vi "diffraction pattern v2.0.vi"() -> ()   [LabVIEW 2019]
doc: "1. before run, set the paramaters on the left of the screen.\n2. flux (magnetic field) is in unit of flux quanta.\n3. Phaserange is in the unit of Pi, the CPR will be build up according to phase range of [-Phaserange/2,Phaserang/2], and such CPR will be a periodic function with Phaserange as period. Enter integer number of multiple times of 4 is preferred.\n4. Use the step setting tab to set resolution of the calculation, you can set how many points is used to define the width of the Josephson junction, how many points to represent the Phaserange\n5. Then you can choose which type of the CPR is used.\n6. Depending on the choose of the CPR, you may want to set the strength of the MBS, \"a\" parameter, the width of the gaussian function used, and the pattern of parity of MBS. Parity pattern has to have same number of elements for positive and negative range.\nEnter the parity 1 or -1 for positive and negative phase +-Pi, +-3Pi, +-5Pi etc.. in to the two arrays.\n7. You can use the index control to read the array elements, then enter the value, you can also delete an element of array by right click, the number of array elements is not limited.\n8. You can change the x,y range, zoom, create cursor etc. to help analyse the plot. Right click to save the data into excel.\n\nEnjoy!\nGuang Yue"
uses:
  dllparameter.ctl
  S-TI-S jj simulation c/Release/ygDLL.dll
panel:
  in  "Tab Control":T1(tab)
  in  "flux start":dbl=-5.0
  in  "flux end":dbl=5.0
  in  "flux step":dbl=0.1
  in  "Geometry steps":i32=201
  in  "Phase steps":i32=201
  in  "CPR Type":T2(ring)
  in  "CPR plot points":i32=500
  in  "parity for negative phase":i32[](array[numeric])=[1, -1, -1, 1]
  in  "Strenth of MBS":dbl=0.5
  in  "parity for positive phase":i32[](array[numeric])=[1, -1, 1, 1]
  in  "Gaussian width":dbl=0.2
  in  "Plot CPR":bool
  in  "Set Noise":bool
  out "Actual flux":dbl
  in  "Flux":dbl
  in  "Plot choice":enum32{"Icp", "Icn"}(radio)
  in  "Geometry Disorder Type":u16(ring) items=["Disorder OFF", "Disorder ON"]
  in  "Plot J vs y":bool
  out "error out":errorcluster
  in  "clear cpr":bool
  in  "clear j":bool
  in  "clearIc":bool
  out "Negative Phase0":dbl
  out "phaserange in Pi":i32=16
  out "Positive Phase0":dbl
  in  "Plot tab":T3(tab)
  out "Diffraction pattern plot":cluster{cluster{dbl, "icn":dbl}[]}[](graph)
  out "Phase0 vs Flux":cluster{cluster{dbl, "icn":dbl}[]}[](graph)
  out "J vs y":cluster{cluster{dbl, "icn":dbl}[]}[](graph)
  out "CPR":cluster{cluster{dbl, "icn":dbl}[]}[](graph)
  in  "Save":bool
  in  "hold":bool=TRUE
  out "Current Flux":dbl=5.0
  out "Remaining steps":i32
  in  "Exit":bool
  in  "Run":bool
  out "Total time s":dbl=5.020437899999706 format="%#_5g"
  in  "stop":bool
  out "Ic negative":dbl=-0.0009989221220817583
  out "Ic positive":dbl=0.000998922122081775 format="%#_5f"
  # "Go to Help menu for instructions, \nor move your mouse cursor on the \nobject for some tip."
  # "Calculate Diffraction pattern"
  # "Version 2.0"
  # "Switch the Tab to choose Plots to save"
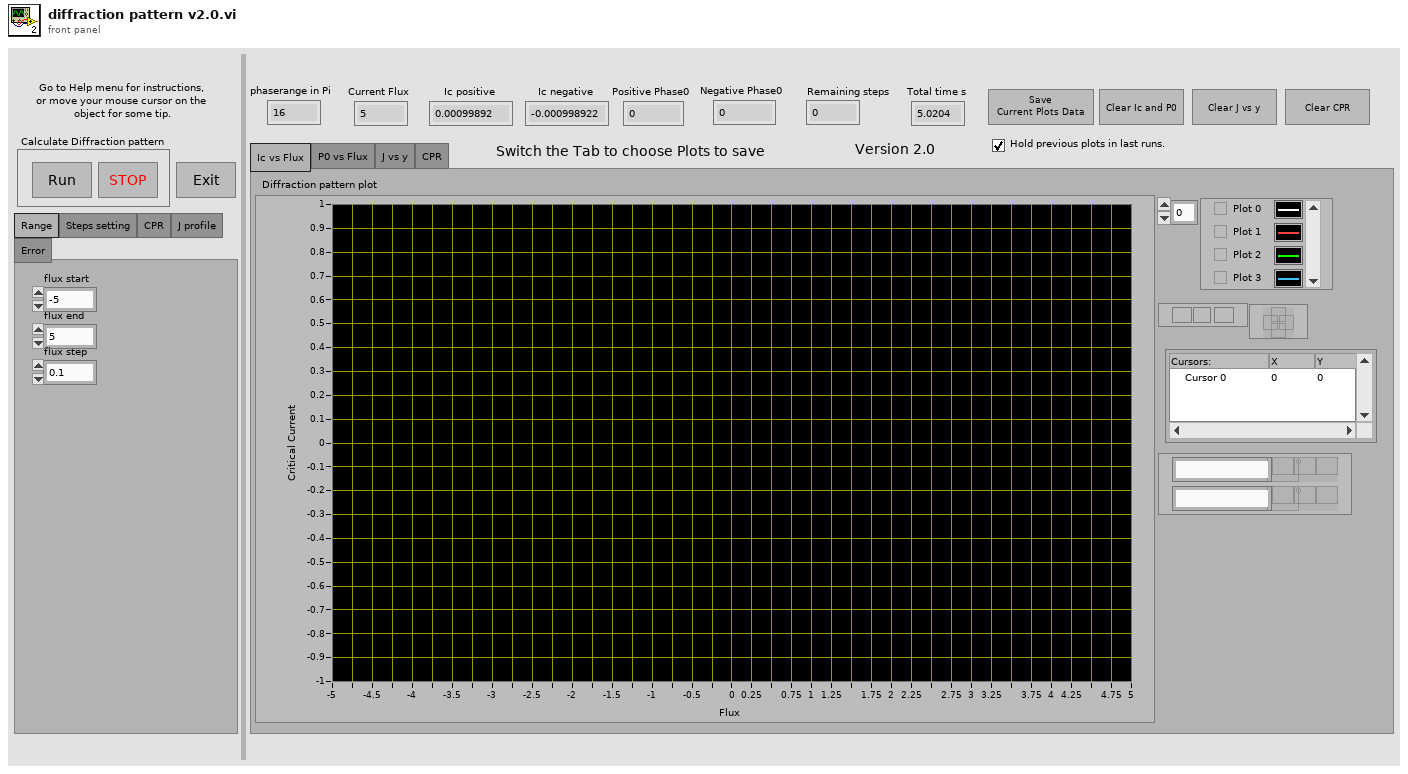
[diagram p1: front panel]
types:
  T1 = enum32{"Range", "Steps setting", "CPR", "J profile", "Error"}
  T2 = enum16{"Regular Josephson effect", "Non-local MBS", "Local MBS same parity", "Local MBS different parity"}
  T3 = enum32{"Ic vs Flux", "P0 vs Flux", "J vs y", "CPR"}
  T4 = enum32{"invalid app kind", "Development System", "Run Time System", "Student Edition", "Embedded LabVIEW", "Evaluation", "Custom"}
  T5 = enum8{"Enabled", "Disabled", "Disabled and Grayed Out"}
  T6 = typedef "dllparameter.ctl" = cluster{"parity for negative phase ":i32[], "parity for positive phase":i32[], "CPR Type":enum16{"Regular Josephson effect", "Non-local MBS", "Local MBS same parity", "Local MBS different parity"}, "Geometry Noise Type":u16, "Geometry steps":i32, "Phase steps":i32, "Strenth of MBS":dbl, "Gaussian width":dbl}
  T7 = cluster{cluster{"phase":dbl, "return type":dbl}[]}
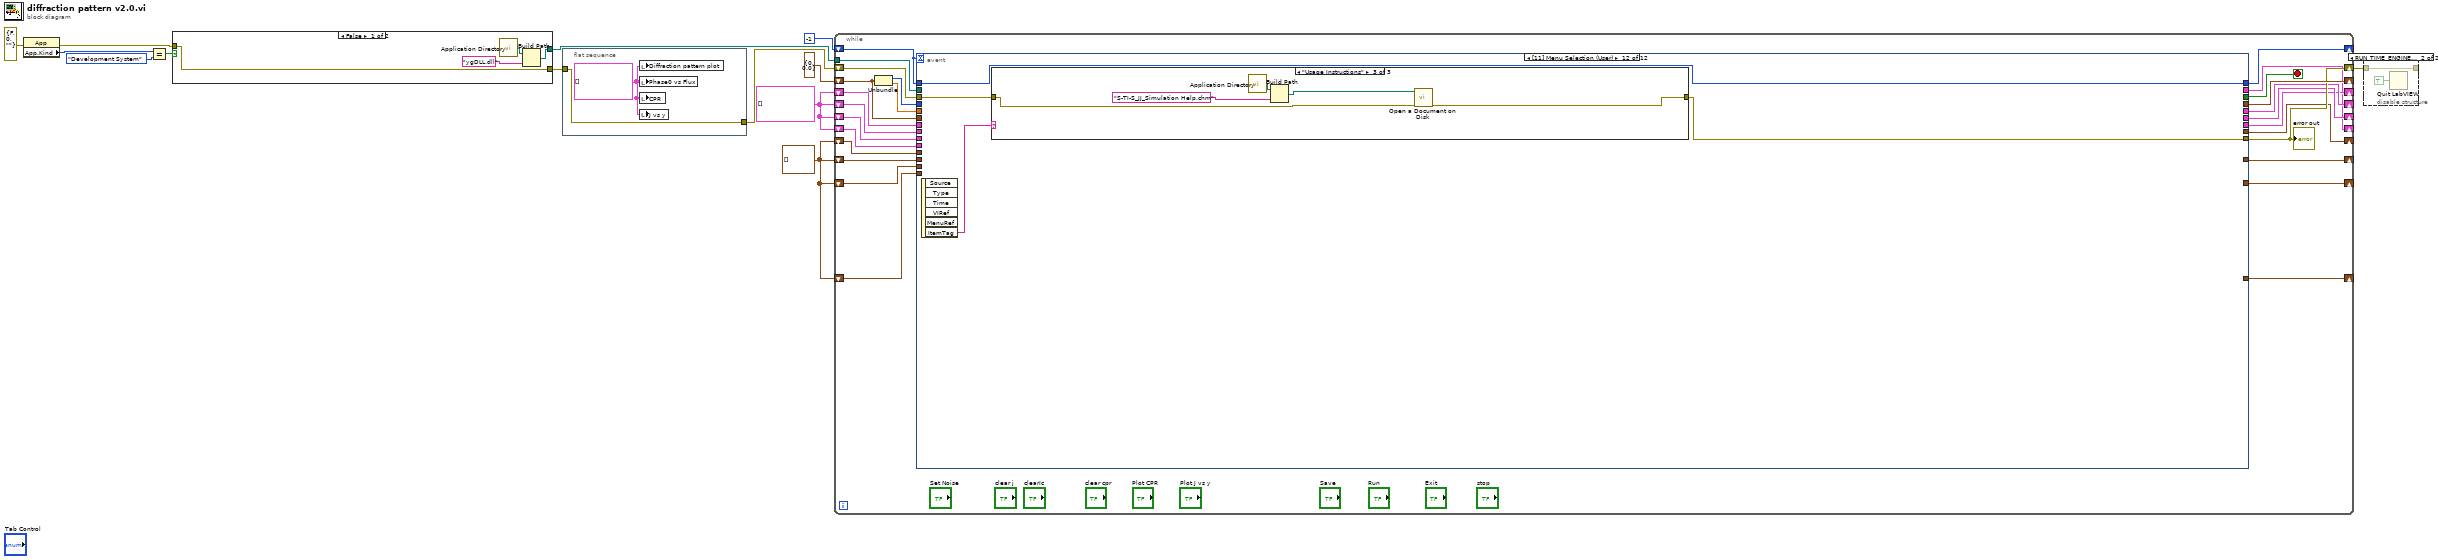
[diagram p0: block diagram]
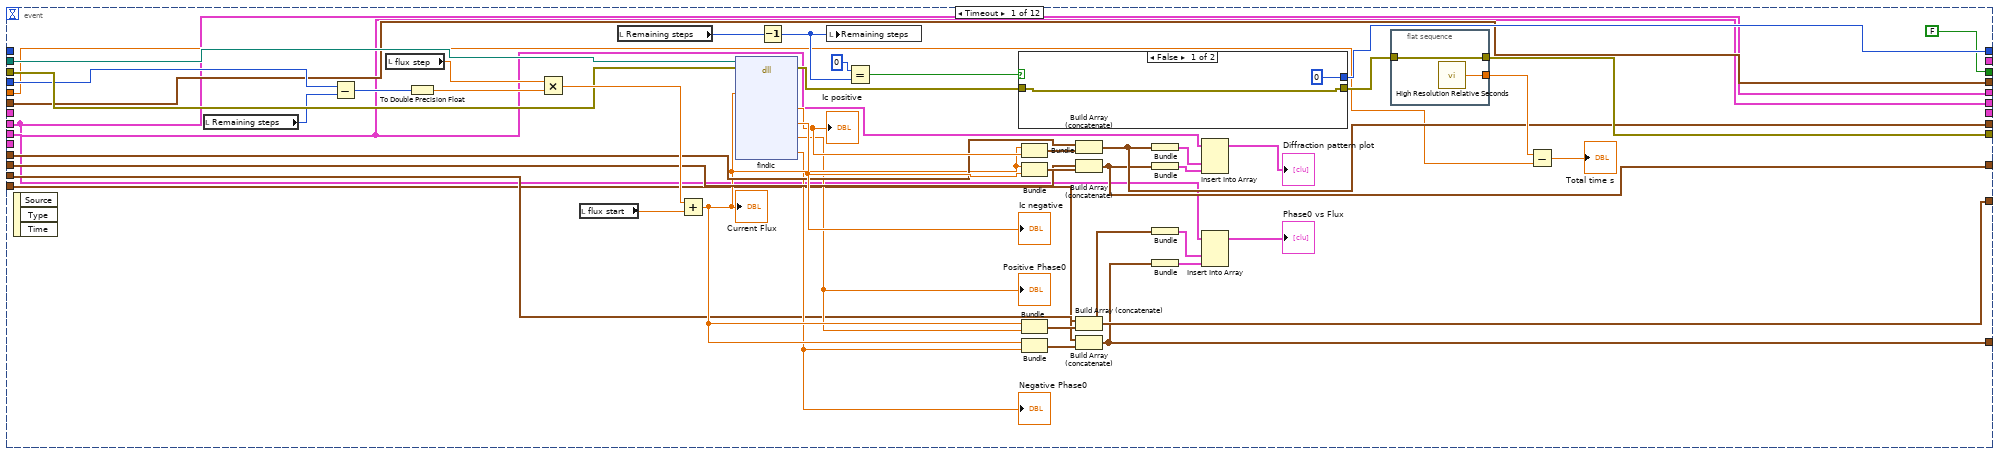
[diagram p3: hidden frame]
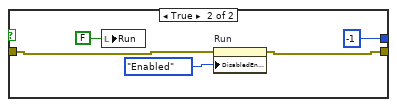
[diagram p4: hidden frame]
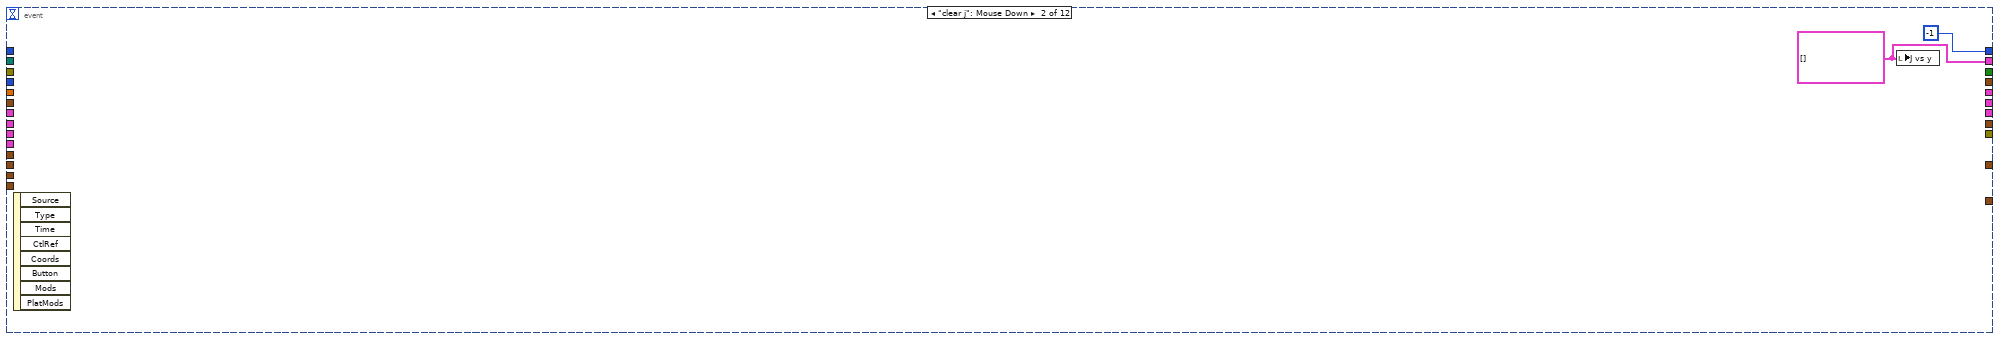
[diagram p5: hidden frame]
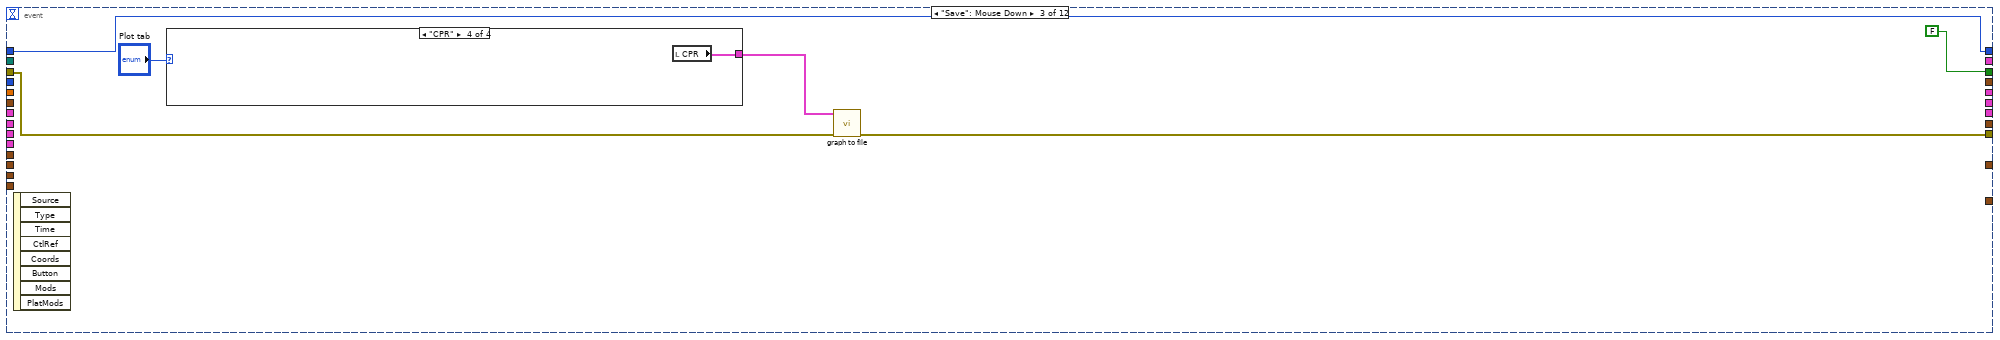
[diagram p6: hidden frame]
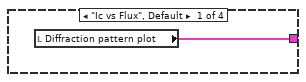
[diagram p7: hidden frame]
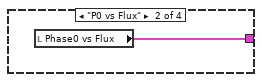
[diagram p8: hidden frame]
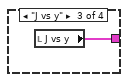
[diagram p9: hidden frame]
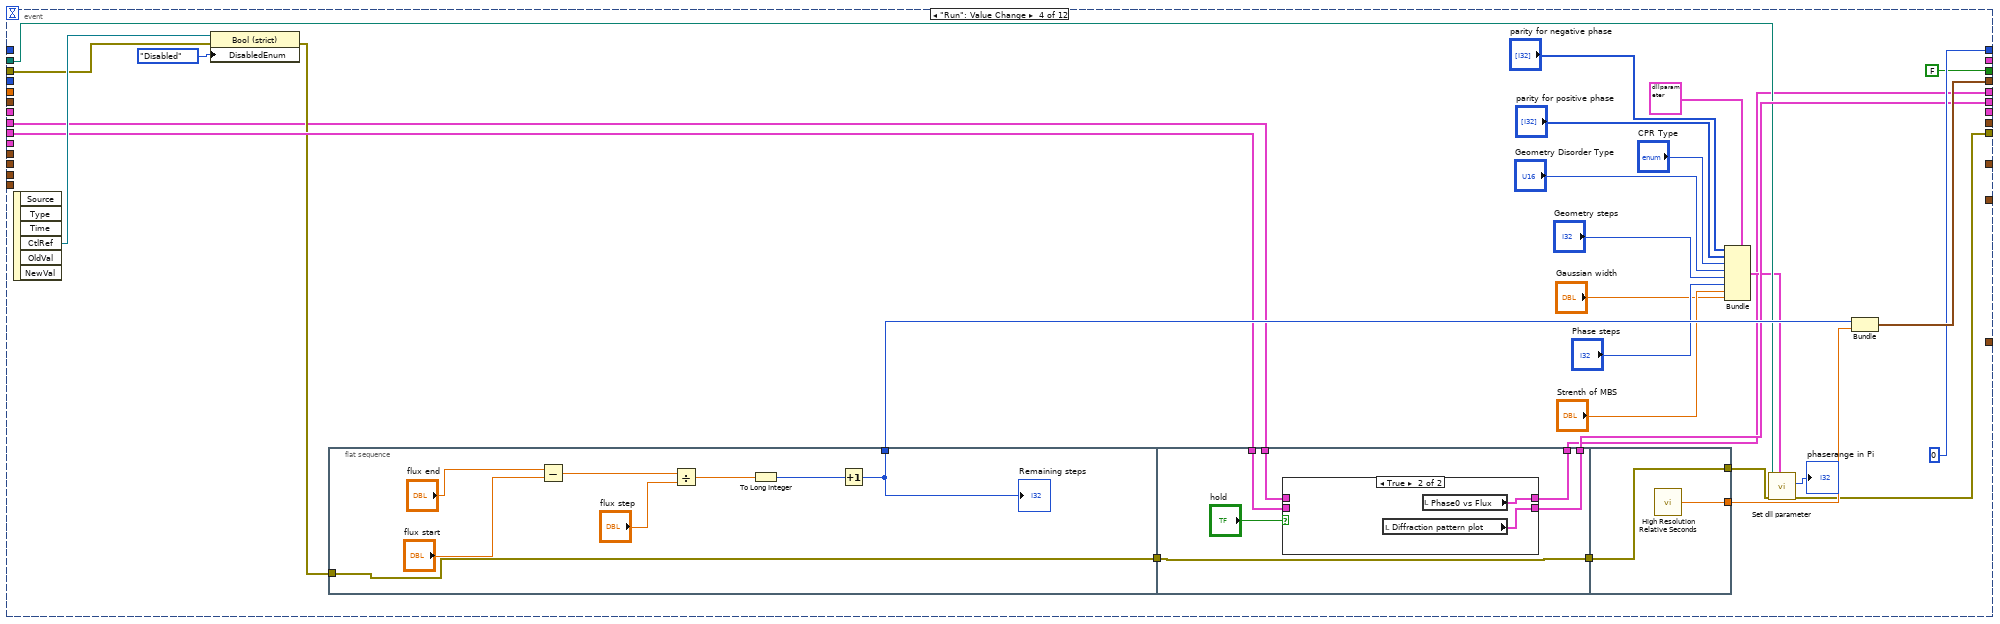
[diagram p10: hidden frame]
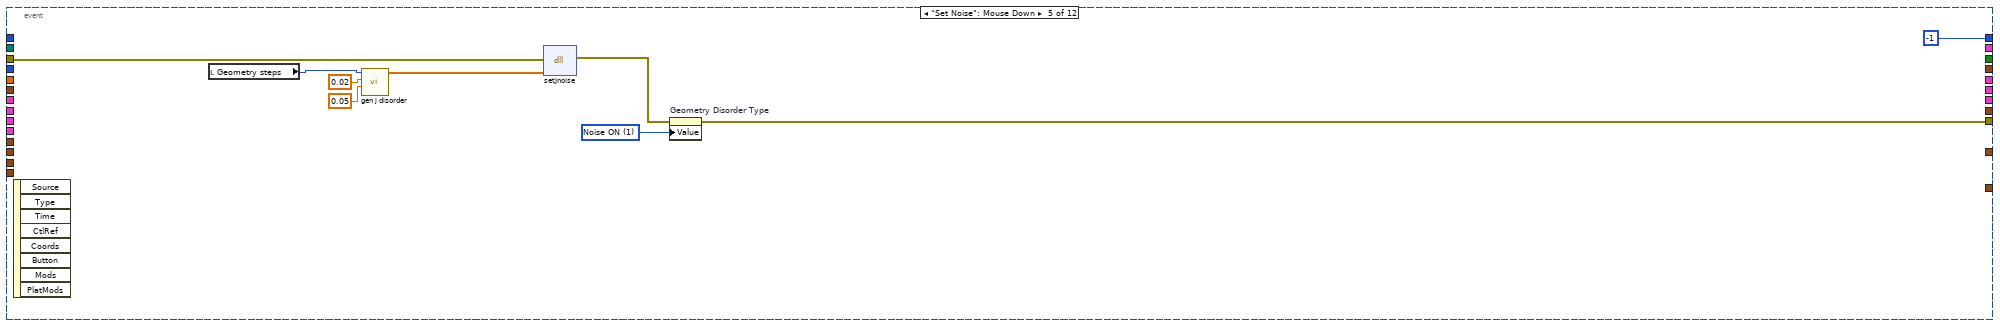
[diagram p12: hidden frame]
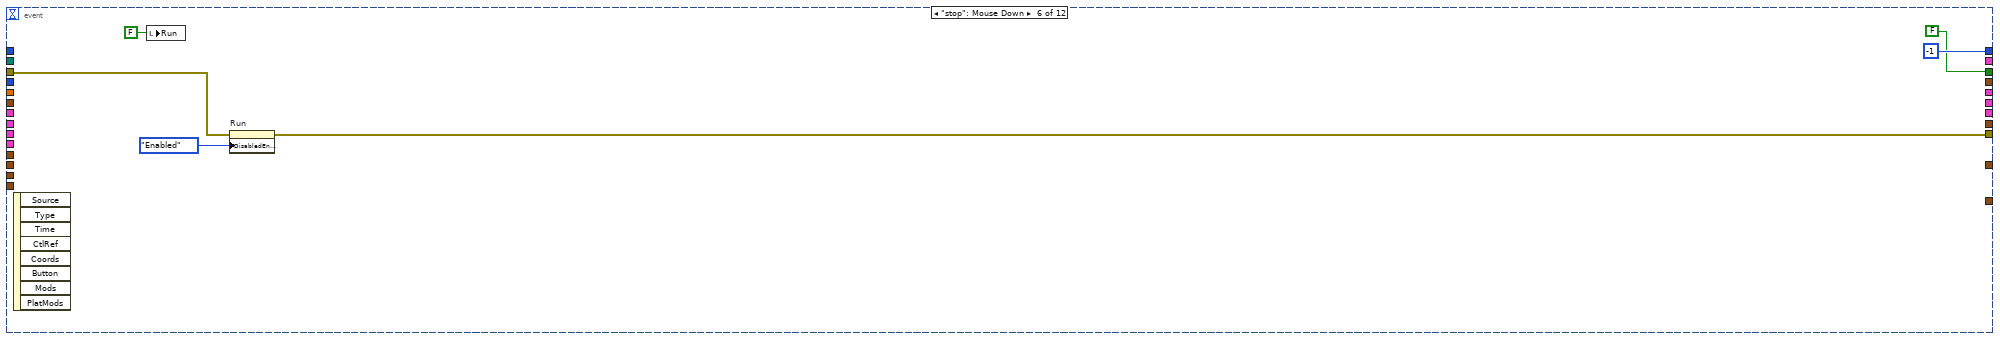
[diagram p13: hidden frame]
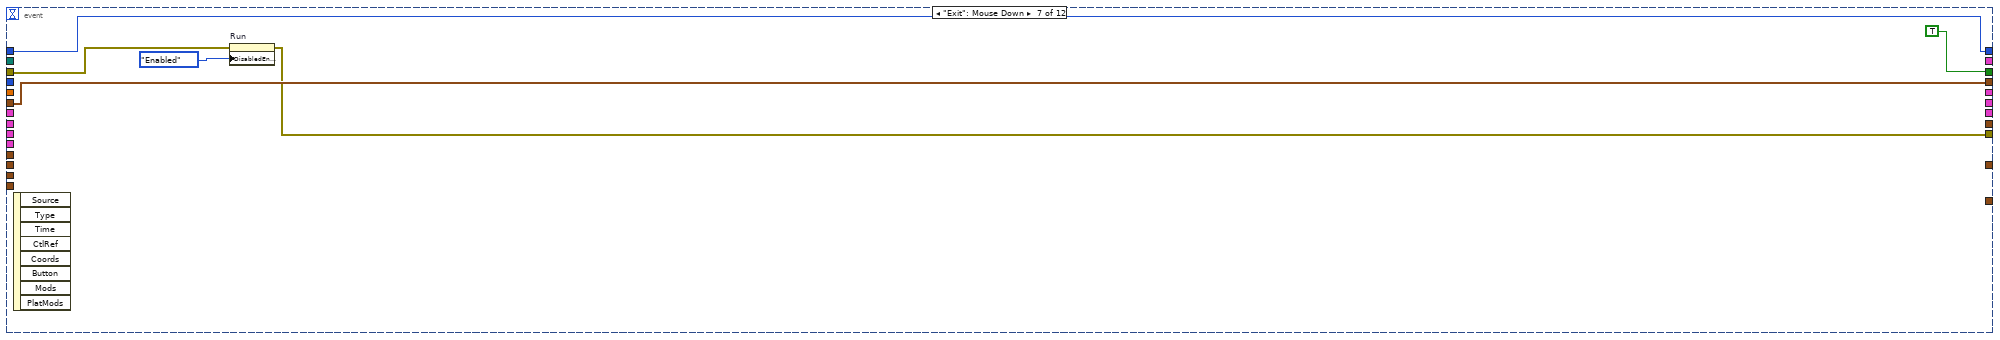
[diagram p14: hidden frame]
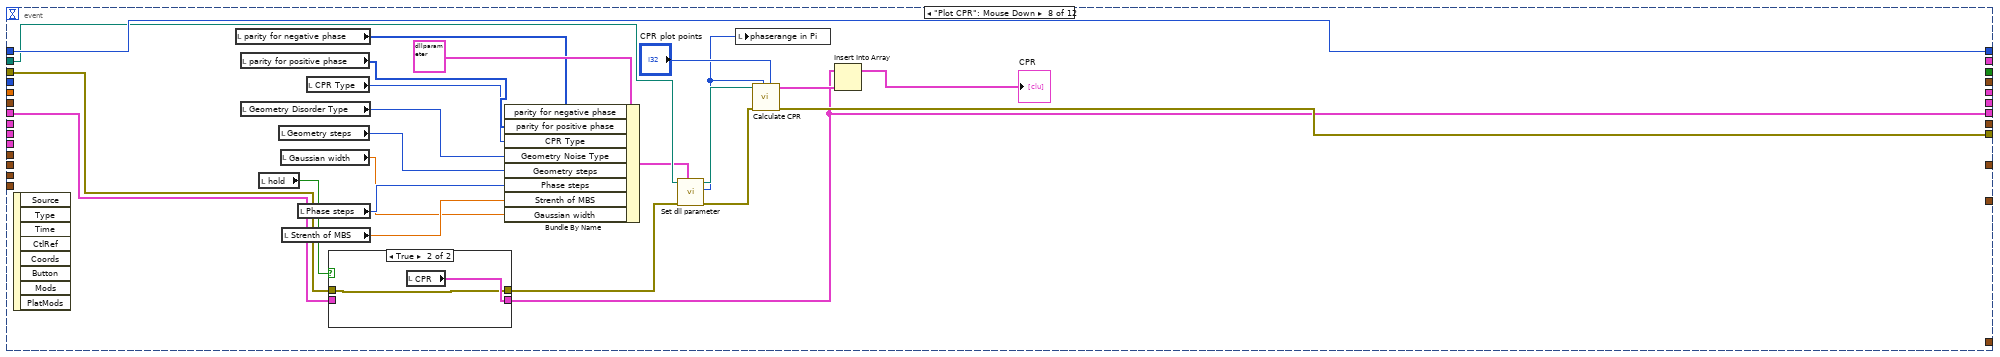
[diagram p15: hidden frame]
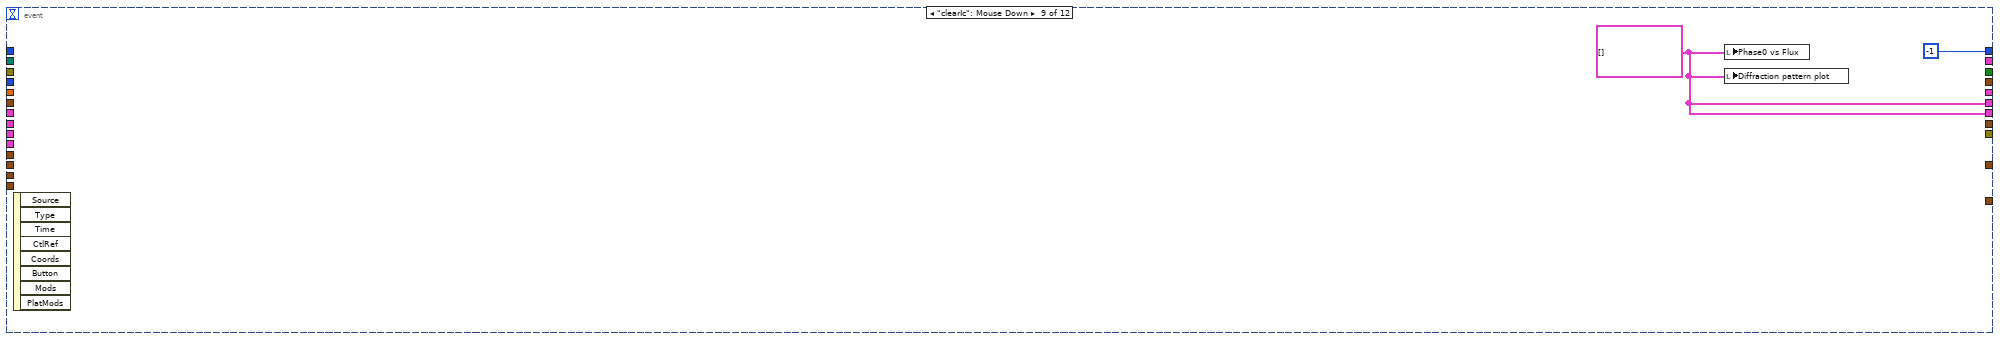
[diagram p17: hidden frame]
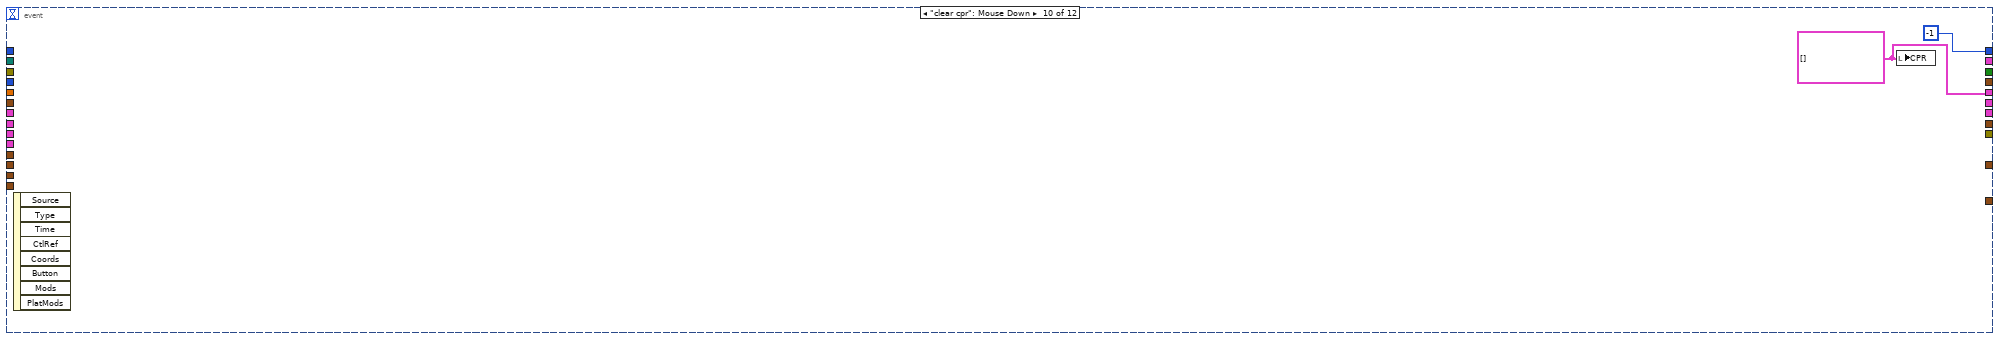
[diagram p18: hidden frame]
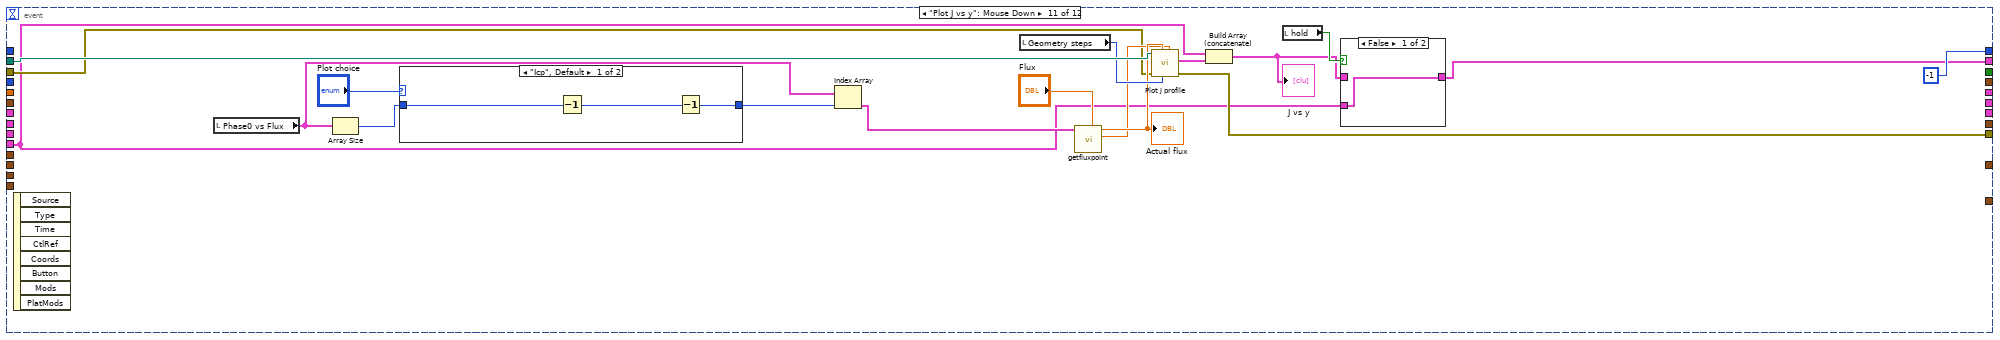
[diagram p19: hidden frame]
diagram:
  w1 = cluster{cluster{dbl, "icn":dbl}[]}[] [] ("appended array")
  w2 = cluster{dbl, "inp":dbl}[] []
  n1 = property class="App"(error in=errorcluster {"status"=FALSE, "code"=0, "source"=""} ("error out")) -> (error out=w9:errorcluster, "App.Kind"=w12:T4)  [unwired: 1 in, 1 out]
  n2 = Equal?(x=w12, y=T4."Development System" ("Application:Kind")) -> (x = y?=w10:bool)
  n3 = case shown="False" w10 {
    tunnel: [w15 path "C:/Users/yg/Box/Guang Yue uiuc research box folder/computation/S-TI-S jj simulation c/Release/ygDLL.dll"] -> w8
    tunnel: w9 -> [w14 w18]
    tunnel: [w14 w18] -> w5
    frame False {
      n4 = call <vilib>:"Application Directory.vi"() -> ("Application Directory"=w17:path)
      n5 = Build Path(base path=w17, name or relative path="ygDLL.dll") -> (appended path=w15:path)
    }
    frame True {
    }
  }
  n6 = flat-sequence {
    tunnel: w5 -> [w21]
    tunnel: [w21] -> w4
    frame #0 {
      w20 = cluster{cluster{dbl, "icn":dbl}[]}[] [] ("appended array")
      n7 = local write "Diffraction pattern plot"(w20) -> ()
      n8 = local write "Phase0 vs Flux"(w20) -> ()
      n9 = local write "CPR"(w20) -> ()
      n10 = local write "J vs y"(w20) -> ()
    }
  }
  n11 = while {
    tunnel: w8 -> [w44]
    shift-right: [w46] -> _
    shift-left: -1 -> [w39]
    shift-right: [w47] -> _
    shift-left: cluster{i32, "relative seconds":dbl} {0, "relative seconds"=0.0} ("output cluster") -> [w40]
    shift-right: [w42] -> w6
    shift-left: w4 -> [w45]
    shift-right: [w37] -> _
    shift-left: w2 -> [w38]
    shift-right: [w36] -> _
    shift-left: w2 -> [w35]
    shift-right: [w32] -> _
    shift-left: w1 -> [w33]
    shift-right: [w29] -> _
    shift-left: w2 -> [w31]
    shift-right: [w28] -> _
    shift-left: w2 -> [w30]
    shift-right: [w26] -> _
    shift-left: w1 -> [w27]
    shift-right: [w24] -> _
    shift-left: w1 -> [w25]
    shift-right: [w22] -> _
    shift-left: w1 -> [w23]
    stop <- w34 stop-if-true
    n12 = Unbundle(w40) -> (w41:i32, "relative seconds"=w43:dbl)
    n13 = event shown="[11] Menu Selection (User)" {
      selector: _ -> [_ _ _ _ _ _ _ _ _ _ _ _]
      dyn-events: _ -> [_ _ _ _ _ _ _ _ _ _ _ _]
      timeout: w39 -> [_ _ _ _ _ _ _ _ _ _ _ _]
      tunnel: [w72 _ _ w140 _ _ w184 _ _ _ _ _] -> w47
      tunnel: [w74 -1 w110 0 -1 -1 w185 w207 -1 -1 -1 w246] -> w46
      tunnel: w45 -> [w87 _ w109 w138 w169 w178 w182 w190 _ _ w221 w245]
      tunnel: w44 -> [w86 _ _ w122 _ _ _ w205 _ _ w234 _]
      tunnel: w43 -> [w61 _ _ _ _ _ _ _ _ _ _ _]
      tunnel: [w85 _ w108 w120 w166 w176 w180 w208 _ _ w224 w244] -> w42
      tunnel: w41 -> [w84 _ _ _ _ _ _ _ _ _ _ _]
      tunnel: w40 -> [w72 _ _ _ _ _ w184 _ _ _ _ _]
      tunnel: w39 -> [_ _ w110 _ _ _ w185 w207 _ _ _ w246]
      tunnel: w38 -> [w69 _ _ _ _ _ _ _ _ _ _ _]
      tunnel: [w70 _ _ _ _ _ _ _ _ _ _ _] -> w37
      tunnel: [w68 _ _ _ _ _ _ _ _ _ _ _] -> w36
      tunnel: w35 -> [w67 _ _ _ _ _ _ _ _ _ _ _]
      tunnel: [FALSE _ FALSE FALSE _ FALSE TRUE _ _ _ _ _] -> w34
      tunnel: w33 -> [w62 _ _ w134 _ _ _ _ _ _ _ _]
      tunnel: [w62 _ _ w135 _ _ _ _ w214 _ _ _] -> w32
      tunnel: w31 -> [w53 _ _ _ _ _ _ _ _ _ _ _]
      tunnel: w30 -> [w52 _ _ _ _ _ _ _ _ _ _ _]
      tunnel: [w51 _ _ _ _ _ _ _ _ _ _ _] -> w29
      tunnel: [w50 _ _ _ _ _ _ _ _ _ _ _] -> w28
      tunnel: w27 -> [w48 _ _ w116 _ _ _ _ _ _ _ _]
      tunnel: [w48 _ _ w117 _ _ _ _ _ w217 _ _] -> w26
      tunnel: w25 -> [_ _ _ _ _ _ _ w188 _ _ _ _]
      tunnel: [_ _ _ _ _ _ _ w186 w214 _ _ _] -> w24
      tunnel: w23 -> [_ _ _ _ _ _ _ _ _ _ w219 _]
      tunnel: [_ w105 _ _ _ _ _ _ _ _ w218 _] -> w22
      event Timeout {
        n14 = event-data() -> ()  [unwired: 1 in, 3 out]
        n15 = local read "Remaining steps"() -> (w83:i32)
        n16 = Subtract(x=w84, y=w83) -> (x-y=w81:i32)
        n17 = local read "flux step"() -> (w82:dbl)
        n18 = To Double Precision Float(number=w81) -> (double precision float=w90:dbl)
        n19 = Multiply(x=w82, y=w90) -> (x*y=w91:dbl)
        n20 = local read "flux start"() -> (w80:dbl)
        n21 = local read "Remaining steps"() -> (w78:i32)
        n22 = Add(x=w91, y=w80) -> (x+y=w56:dbl)
        "Current Flux" <- w56
        n23 = dll-call lib="C:/Users/yg/Box/Guang Yue uiuc research box folder/computation/S-TI-S jj simulation c/Release/ygDLL.dll" fn="findIc"(path in=w86, error in=w87, "flux"=w56) -> (error out=w79:errorcluster, "inp"=w92:dbl, "icn"=w93:dbl, "pp0"=w55:dbl, "pn0"=w54:dbl)  [unwired: 7 in, 1 out]
        "Ic positive" <- w92
        "Ic negative" <- w93
        "Positive Phase0" <- w55
        "Negative Phase0" <- w54
        n24 = Decrement(x=w78) -> (x-1=w76:i32)
        n25 = local write "Remaining steps"(w76) -> ()
        n26 = Equal?(x=0, y=w76) -> (x = y?=w75:bool)
        n27 = case shown="False" w75 {
          tunnel: w79 -> [w95 w100]
          tunnel: [0 -1] -> w74
          tunnel: [w95 w99] -> w73
          frame False {
          }
          frame True {
            n28 = local write "Run"(FALSE ("Run")) -> ()
            n29 = property on="Run" class="Bool (strict)"(error in=w100, "DisabledEnum"=T5."Enabled" ("Disabled")) -> (error out=w99:errorcluster)  [unwired: 1 in, 1 out]
          }
        }
        n30 = Bundle(w56, "inp"=w92) -> (w71:cluster{dbl, "inp":dbl})  [unwired: 1 in]
        n31 = Bundle(w56, "icn"=w93) -> (w94:cluster{dbl, "icn":dbl})  [unwired: 1 in]
        n32 = Bundle(w56, "pp0"=w55) -> (w59:cluster{dbl, "pp0":dbl})  [unwired: 1 in]
        n33 = Bundle(w56, "pn0"=w54) -> (w60:cluster{dbl, "pn0":dbl})  [unwired: 1 in]
        n34 = Build Array (concatenate)(w69, w71) -> (w70:cluster{dbl, "inp":dbl}[])
        n35 = Build Array (concatenate)(w67, w94) -> (w68:cluster{dbl, "icn":dbl}[])
        n36 = Build Array (concatenate)(w53, w59) -> (w51:cluster{dbl, "pp0":dbl}[])
        n37 = Build Array (concatenate)(w52, w60) -> (w50:cluster{dbl, "pn0":dbl}[])
        n38 = Bundle(w70) -> (w65:cluster{cluster{dbl, "inp":dbl}[]})  [unwired: 1 in]
        n39 = Bundle(w68) -> (w64:cluster{cluster{dbl, "icn":dbl}[]})  [unwired: 1 in]
        n40 = Bundle(w51) -> (w58:cluster{cluster{dbl, "pp0":dbl}[]})  [unwired: 1 in]
        n41 = Bundle(w50) -> (w57:cluster{cluster{dbl, "pn0":dbl}[]})  [unwired: 1 in]
        n42 = Insert Into Array(array=w62, new element #1=w65, new element #2=w64) -> (→"Diffraction pattern plot":cluster{cluster{dbl, "icn":dbl}[]}[])  [unwired: 1 in]
        n43 = Insert Into Array(array=w48, new element #1=w58, new element #2=w57) -> (→"Phase0 vs Flux":cluster{cluster{dbl, "icn":dbl}[]}[])  [unwired: 1 in]
        n44 = flat-sequence {
          tunnel: w73 -> [w103]
          tunnel: [w103] -> w85
          tunnel: [w102] -> w89
          frame #0 {
            n45 = call <vilib>:"High Resolution Relative Seconds.vi"() -> ("relative seconds"=w102:dbl)
          }
        }
        n46 = Subtract(x=w89, y=w61) -> (x-y=→"Total time s":dbl)
      }
      event "clear j": Mouse Down {
        w105 = cluster{cluster{dbl, "return type":dbl}[]}[] [] ("appended array")
        n47 = event-data() -> ()  [unwired: 1 in, 8 out]
        n48 = local write "J vs y"(w105) -> ()
      }
      event "Save": Mouse Down {
        n49 = event-data() -> ()  [unwired: 1 in, 8 out]
        n50 = case shown="\"CPR\"" "Plot tab" {
          tunnel: [w112 w113 w114 w115] -> w106
          frame "Ic vs Flux", Default {
            n51 = local read "Diffraction pattern plot"() -> (w112:cluster{cluster{dbl, "icn":dbl}[]}[])
          }
          frame "P0 vs Flux" {
            n52 = local read "Phase0 vs Flux"() -> (w113:cluster{cluster{dbl, "icn":dbl}[]}[])
          }
          frame "J vs y" {
            n53 = local read "J vs y"() -> (w114:cluster{cluster{dbl, "icn":dbl}[]}[])
          }
          frame "CPR" {
            n54 = local read "CPR"() -> (w115:cluster{cluster{dbl, "icn":dbl}[]}[])
          }
        }
        n55 = call "graph to file.vi"("error in (no error)"=w109, "Input array"=w106) -> ("error out"=w108:errorcluster)  [unwired: 9 in]
      }
      event "Run": Value Change {
        n56 = event-data() -> ("CtlRef"=w144:refnum<vi>)  [unwired: 1 in, 5 out]
        n57 = property class="Bool (strict)"(reference=w144, error in=w138, "DisabledEnum"=T5."Disabled" ("Disabled")) -> (error out=w133:errorcluster)  [unwired: 1 out]
        n58 = flat-sequence {
          tunnel: w133 -> [w146]
          tunnel: [w145] -> w142
          tunnel: [w146] -> w132
          tunnel: w132 -> [w158]
          tunnel: [w158] -> w136
          tunnel: [w156] -> w135
          tunnel: w134 -> [w155]
          tunnel: [w154] -> w117
          tunnel: w116 -> [w153]
          tunnel: [w164] -> w123
          tunnel: w136 -> [w164]
          tunnel: [w163] -> w141
          frame #0 {
            n59 = Subtract(x="flux end", y="flux start") -> (x-y=w151:dbl)
            n60 = Divide(x=w151, y="flux step") -> (x/y=w150:dbl)
            n61 = To Long Integer(number=w150) -> (32bit integer=w149:i32)
            n62 = Increment(x=w149) -> (x+1=w145:i32)
            "Remaining steps" <- w145
          }
          frame #1 {
            n63 = case shown="True" "hold" {
              tunnel: [w160 w162] -> w156
              tunnel: w155 -> [w160 _]
              tunnel: [w159 w161] -> w154
              tunnel: w153 -> [w159 _]
              frame False {
              }
              frame True {
                n64 = local read "Diffraction pattern plot"() -> (w162:cluster{cluster{dbl, "icn":dbl}[]}[])
                n65 = local read "Phase0 vs Flux"() -> (w161:cluster{cluster{dbl, "icn":dbl}[]}[])
              }
            }
          }
          frame #2 {
            n66 = call <vilib>:"High Resolution Relative Seconds.vi"() -> ("relative seconds"=w163:dbl)
          }
        }
        n67 = Bundle(cluster=T6 {"parity for negative phase "=[], "parity for positive phase"=[], "CPR Type"=enum."Regular Josephson effect", "Geometry Noise Type"=0, "Geometry steps"=0, "Phase steps"=0, "Strenth of MBS"=0.0, "Gaussian width"=0.0} ("output cluster"), "parity for negative phase"="parity for negative phase", "parity for positive phase"="parity for positive phase", "CPR Type"="CPR Type", "Geometry Noise Type"="Geometry Disorder Type", "Geometry steps"="Geometry steps", "Phase steps"="Phase steps", "Strenth of MBS"="Strenth of MBS", "Gaussian width"="Gaussian width") -> (w121:T6)
        n68 = call "Set dll parameter.vi"("output cluster"=w121, "error in (no error)"=w123, "path in"=w122) -> ("error out"=w120:errorcluster, "phaserange in Pi"=→"phaserange in Pi":i32)  [unwired: 6 in, 1 out]
        n69 = Bundle(w142, "relative seconds"=w141) -> (w140:cluster{i32, "relative seconds":dbl})  [unwired: 1 in]
      }
      event "Set Noise": Mouse Down {
        w165 = u16 1 items=["Noise OFF", "Noise ON"] ("Geometry Noise Type")
        n70 = event-data() -> ()  [unwired: 1 in, 8 out]
        n71 = local read "Geometry steps"() -> (w172:i32)
        n72 = call "gen j disorder.vi"("Step width"=0.05, "App"=0.02, "Points"=w172) -> ("Array"=w168:dbl[])  [unwired: 8 in]
        n73 = dll-call lib="C:/Users/yg/Box/Guang Yue uiuc research box folder/computation/S-TI-S jj simulation c/Release/ygDLL.dll" fn="setJnoise"(error in=w169, "arg1"=w168) -> (error out=w167:errorcluster)  [unwired: 4 in, 1 out]
        n74 = property on="Geometry Disorder Type" class="Ring (strict)"(error in=w167, "Value"=w165) -> (error out=w166:errorcluster)  [unwired: 1 in, 1 out]
      }
      event "stop": Mouse Down {
        n75 = event-data() -> ()  [unwired: 1 in, 8 out]
        n76 = local write "Run"(FALSE ("Run")) -> ()
        n77 = property on="Run" class="Bool (strict)"(error in=w178, "DisabledEnum"=T5."Enabled" ("Disabled")) -> (error out=w176:errorcluster)  [unwired: 1 in, 1 out]
      }
      event "Exit": Mouse Down {
        n78 = event-data() -> ()  [unwired: 1 in, 8 out]
        n79 = property on="Run" class="Bool (strict)"(error in=w182, "DisabledEnum"=T5."Enabled" ("Disabled")) -> (error out=w180:errorcluster)  [unwired: 1 in, 1 out]
      }
      event "Plot CPR": Mouse Down {
        n80 = event-data() -> ()  [unwired: 1 in, 8 out]
        n81 = local read "parity for negative phase"() -> (w201:i32[])
        n82 = local read "parity for positive phase"() -> (w200:i32[])
        n83 = local read "Geometry Disorder Type"() -> (w198:u16)
        n84 = local read "hold"() -> (w191:bool)
        n85 = local read "Geometry steps"() -> (w197:i32)
        n86 = local read "Gaussian width"() -> (w194:dbl)
        n87 = local read "Strenth of MBS"() -> (w195:dbl)
        n88 = local read "Phase steps"() -> (w196:i32)
        n89 = local read "CPR Type"() -> (w199:T2)
        n90 = case shown="True" w191 {
          tunnel: [w211 w212] -> w189
          tunnel: w190 -> [w211 w212]
          tunnel: [w210 w213] -> w186
          tunnel: w188 -> [w210 _]
          frame False {
          }
          frame True {
            n91 = local read "CPR"() -> (w213:cluster{cluster{dbl, "icn":dbl}[]}[])
          }
        }
        n92 = Bundle By Name(cluster=T6 {"parity for negative phase "=[], "parity for positive phase"=[], "CPR Type"=enum."Regular Josephson effect", "Geometry Noise Type"=0, "Geometry steps"=0, "Phase steps"=0, "Strenth of MBS"=0.0, "Gaussian width"=0.0} ("output cluster"), "parity for negative phase"=w201, "parity for positive phase"=w200, "CPR Type"=w199, "Geometry Noise Type"=w198, "Geometry steps"=w197, "Phase steps"=w196, "Strenth of MBS"=w195, "Gaussian width"=w194) -> (w202:T6)
        n93 = call "Set dll parameter.vi"("output cluster"=w202, "error in (no error)"=w189, "path in"=w205) -> ("error out"=w206:errorcluster, "phaserange in Pi"=w193:i32, "path out"=w204:path)  [unwired: 6 in]
        n94 = local write "phaserange in Pi"(w193) -> ()
        n95 = call "Calculate CPR.vi"("steps"="CPR plot points", "phase range"=w193, "error in (no error)"=w206, "path in"=w204) -> ("error out"=w208:errorcluster, "output Plot"=w192:T7)  [unwired: 6 in]
        n96 = Insert Into Array(array=w186, new element=w192) -> (→"CPR":cluster{cluster{dbl, "icn":dbl}[]}[])  [unwired: 1 in]
      }
      event "clearIc": Mouse Down {
        w214 = cluster{cluster{dbl, "icn":dbl}[]}[] [] ("CPR")
        n97 = event-data() -> ()  [unwired: 1 in, 8 out]
        n98 = local write "Phase0 vs Flux"(w214) -> ()
        n99 = local write "Diffraction pattern plot"(w214) -> ()
      }
      event "clear cpr": Mouse Down {
        w217 = cluster{cluster{dbl, "icn":dbl}[]}[] [] ("Phase0 vs Flux")
        n100 = event-data() -> ()  [unwired: 1 in, 8 out]
        n101 = local write "CPR"(w217) -> ()
      }
      event "Plot J vs y": Mouse Down {
        n102 = event-data() -> ()  [unwired: 1 in, 8 out]
        n103 = local read "Phase0 vs Flux"() -> (w232:cluster{cluster{dbl, "icn":dbl}[]}[])
        n104 = Array Size(array=w232) -> (size(s)=w230:i32)
        n105 = case shown="\"Icp\", Default" "Plot choice" {
          tunnel: w230 -> [w240 w242]
          tunnel: [w239 w241] -> w229
          frame "Icp", Default {
            n106 = Decrement(x=w240) -> (x-1=w238:i32)
            n107 = Decrement(x=w238) -> (x-1=w239:i32)
          }
          frame "Icn" {
            n108 = Decrement(x=w242) -> (x-1=w241:i32)
          }
        }
        n109 = Index Array(array=w232, index=w229) -> (element=w228:cluster{cluster{dbl, "icn":dbl}[]})
        n110 = local read "Geometry steps"() -> (w233:i32)
        n111 = call "getfluxpoint.vi"("flux"="Flux", "Plot"=w228) -> ("phase0"=w225:dbl, "actual flux"=w226:dbl)  [unwired: 8 in]
        "Actual flux" <- w226
        n112 = call "Plot J profile.vi"("p0"=w225, "Steps"=w233, "flux"=w226, "error in (no error)"=w221, "path in"=w234) -> ("error out"=w224:errorcluster, "plot"=w223:cluster{cluster{dbl, "return type":dbl}[]})  [unwired: 4 in, 1 out]
        n113 = Build Array (concatenate)(w219, w223) -> (w220:cluster{cluster{dbl, "return type":dbl}[]}[])
        "J vs y" <- w220
        n114 = local read "hold"() -> (w222:bool)
        n115 = case shown="False" w222 {
          tunnel: w220 -> [_ w237]
          tunnel: [w236 w237] -> w218
          tunnel: w219 -> [w236 _]
          frame False {
          }
          frame True {
          }
        }
      }
      event Menu Selection (User) {
        n116 = event-data() -> ("ItemTag"=w243:string)  [unwired: 1 in, 5 out]
        n117 = case shown="\"Usage Instructions\"" w243 {
          tunnel: w245 -> [w247 w249 w253]
          tunnel: [w247 w248 w251] -> w244
          frame Default {
          }
          frame "About_me" {
            n118 = call "About this program"("error in (no error)"=w249, "Message"="This software is developed for simulation on S-TI-S Josephson junction. Majorana Bound State, iregular current phase relation are considered. The calucation results include diffraction pattern, optimised phase0, current phase relation plot, local current distribution etc.\nChange Log: \nv1.0 basic program for diffraction pattern simulation\nv1.6 Added multi-plots feature and easy data save function.\nv 2.0 Add calculation of current phase relation, optimised phase0, plot of local current. Geometry disorder on the current density along y direction.\nGuang Yue, DVH group") -> ("error out"=w248:errorcluster)  [unwired: 8 in, 1 out]
          }
          frame "Usage Instructions" {
            n119 = call <vilib>:"Application Directory.vi"() -> ("Application Directory"=w255:path)
            n120 = Build Path(base path=w255, name or relative path="S-TI-S_JJ_Simulation Help.chm") -> (appended path=w252:path)
            n121 = call <vilib>:"Open a Document on Disk.vi"("error in (no error)"=w253, "document path"=w252) -> ("error out"=w251:errorcluster)  [unwired: 5 in]
          }
        }
      }
    }
    "error out" <- w42
  }
  n122 = disable-structure shown="RUN_TIME_ENGINE==True" {
    disable-tunnel: [w256 w257] -> _
    disable-tunnel: w6 -> [w256 w257]
    frame condition #0 (active) {
    }
    frame condition #1 {
      n123 = Quit LabVIEW(quit? (T)=TRUE) -> ()
    }
  }
